vi "getSubArray2D.vi"(8 "error in (no error)":errorcluster, 9 "Index Array Cluster":T1, 11 "2D Array":dbl[][](array[numeric])) -> (0 "error out":errorcluster, 3 "Sub-Array":dbl[][](array[numeric]))   [LabVIEW 2016]
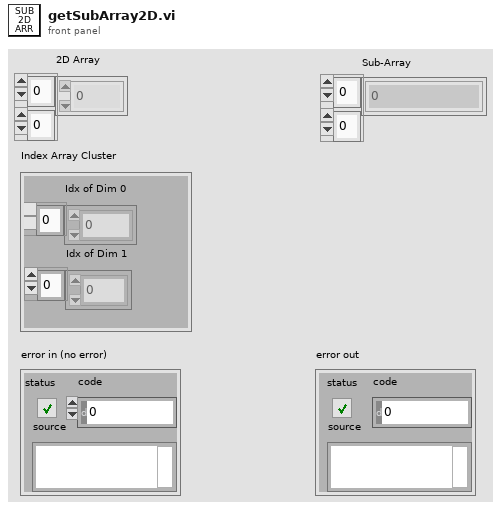
[diagram p1: front panel]
types:
  T1 = cluster{"Idx of Dim 0":i32[], "Idx of Dim 1":i32[]}
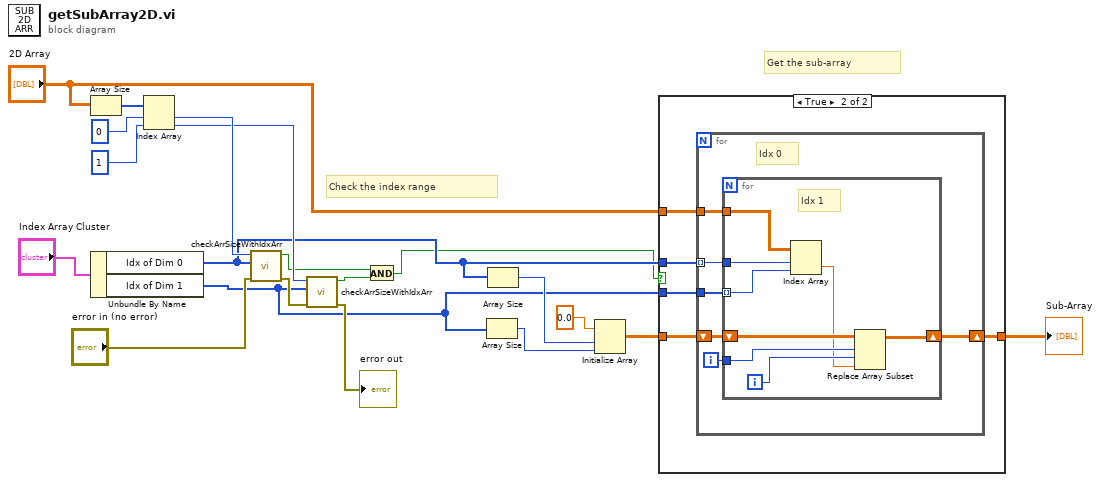
[diagram p0: block diagram]
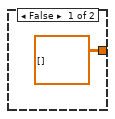
[diagram p2: hidden frame]
diagram:
  # "Check the index range"
  # "Get the sub-array"
  n1 = Array Size(array="2D Array") -> (size(s)=w13:i32[])
  n2 = Unbundle By Name("Index Array Cluster") -> ("Idx of Dim 0"=w3:i32[], "Idx of Dim 1"=w2:i32[])
  n3 = Index Array(array=w13, index #1=0 ("index"), index #2=1 ("index")) -> (element #1=w10:i32, element #2=w9:i32)
  n4 = call "checkArrSizeWithIdxArr.vi"("error in (no error)"="error in (no error)", "Idx Array"=w3, "Array Size"=w10) -> ("error out"=w7:errorcluster, "In Spec"=w5:bool)  [unwired: 7 in]
  n5 = call "checkArrSizeWithIdxArr.vi"("error in (no error)"=w7, "Idx Array"=w2, "Array Size"=w9) -> ("error out"=→"error out":errorcluster, "In Spec"=w4:bool)  [unwired: 7 in]
  n6 = And(x=w5, y=w4) -> (x .and. y?=w1:bool)
  n7 = Array Size(array=w2) -> (size(s)=w17:i32)
  n8 = Array Size(array=w3) -> (size(s)=w18:i32)
  n9 = Initialize Array(0.0 ("element"), w18, w17) -> (w19:dbl[][])
  n10 = case shown="True" w1 {
    tunnel: w19 -> [_ w26]
    tunnel: [dbl[][] [] w25] -> w16
    tunnel: "2D Array" -> [_ w24]
    tunnel: w3 -> [_ w23]
    tunnel: w2 -> [_ w22]
    frame False {
    }
    frame True {
      n11 = for {
        shift-right: [w28] -> w25
        shift-left: w26 -> [w29]
        tunnel: w23 -> [w32] mode=indexing
        tunnel: w22 -> [w31]
        tunnel: w24 -> [w30]
        i -> [w27]
        # "Idx 0"
        n12 = for {
          shift-right: [w36] -> w28
          shift-left: w29 -> [w37]
          tunnel: w32 -> [w39]
          tunnel: w31 -> [w38] mode=indexing
          tunnel: w30 -> [w40]
          tunnel: w27 -> [w35]
          i -> [w34]
          # "Idx 1"
          n13 = Index Array(array=w40, index (row)=w39, index (col)=w38) -> (element=w33:dbl)
          n14 = Replace Array Subset(array=w37, new element=w33, index (row)=w35, index (col)=w34) -> (w36:dbl[][])
        }
      }
    }
  }
  "Sub-Array" <- w16
